vi "parse problem 1.vi"() -> ()   [LabVIEW 2010]
uses:
  <vilib>/xml/NI_XML.lvlib
panel:
  out "node text":string
  in  "XPath expression":string
  in  "XML string":string
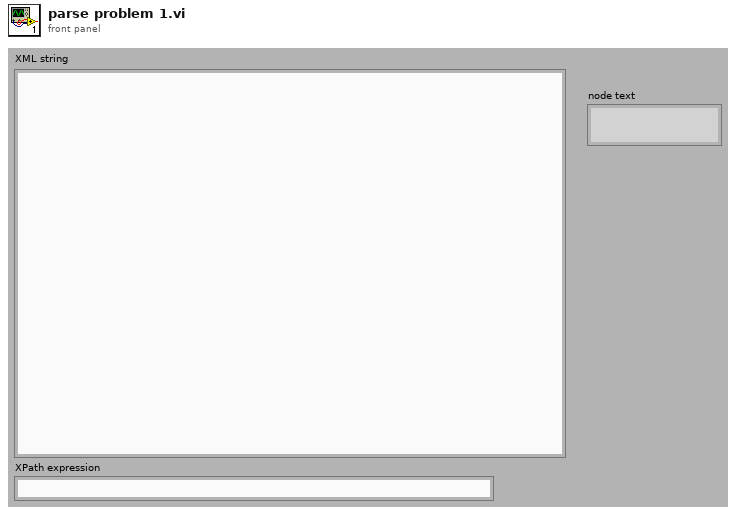
[diagram p1: front panel]
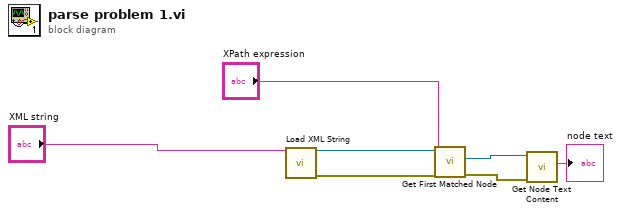
[diagram p0: block diagram]
diagram:
  n1 = call <vilib>:"Load XML String.vi"("XML string"="XML string") -> ("DOM document out"=w4:refnum<k20>, "error out"=w5:errorcluster)  [unwired: 1 in, 12 out]
  n2 = call <vilib>:"Get First Matched Node.vi"("error in (no error)"=w5, "XPath expression"="XPath expression", "node in"=w4) -> ("error out"=w6:errorcluster, "node result"=w7:refnum<k20>)  [unwired: 6 in, 1 out]
  n3 = call <vilib>:"Get Node Text Content.vi"("error in (no error)"=w6, "node in"=w7) -> ("node text"=→"node text":string)  [unwired: 7 in, 2 out]
